vi "LinxDigitalRead.vi"(8 "Error In":errorcluster, 10 "Channels":u8[](array[numeric]), 11 "LINX Resource":T1) -> (0 "Error Out":errorcluster, 2 "Values":bool[](array[boolean]), 3 "LINX Resource":T1)   [LabVIEW 2020, in "LMH-LINX.lvlib" / "Local IO.lvlib"]
uses:
  Local IO.lvlib
  Type Defs/LINX Ref.ctl
  Type Defs/Platform.ctl
  Type Defs/Interface.ctl
  Device/Type Defs/LINX Device Config.ctl
  Device/Type Defs/TCP Config.ctl
  Device/Type Defs/Channels.ctl
  <vilib>/MakerHub/LINX/Resources/liblinxdevice.dll
  LMH-LINX.lvlib
  Device/Device.lvlib
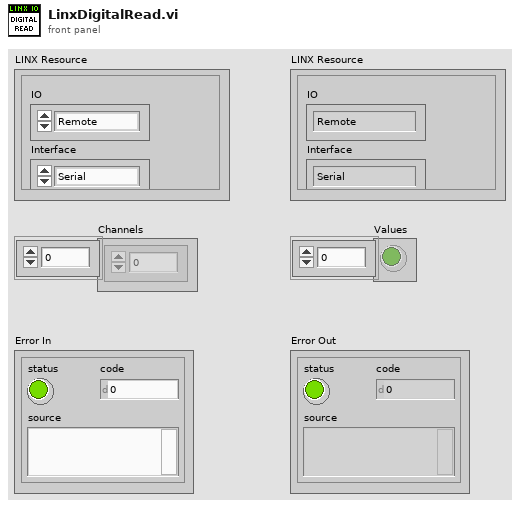
[diagram p1: front panel]
types:
  T1 = typedef "LMH-LINX.lvlib/LINX Ref.ctl" = cluster{"IO":T2, "Interface":T3, "LINX Device Config":T4}
  T2 = typedef "LMH-LINX.lvlib/Platform.ctl" = enum16{"Remote", "Local"}
  T3 = typedef "LMH-LINX.lvlib/Interface.ctl" = enum16{"Serial", "TCP"}
  T4 = typedef "LMH-LINX.lvlib/Device.lvlib/LINX Device Config.ctl" = cluster{"Interface":T3, "COM Port":refnum<visa-resource-name>, "TCP Configuration":T5, "Device Family":u8, "Device ID":u8, "Device Name":string, "TCP Ref":refnum<k5>, "Channels":T6}
  T5 = typedef "LMH-LINX.lvlib/Device.lvlib/TCP Config.ctl" = cluster{"IP Address":string, "Port":u16}
  T6 = typedef "LMH-LINX.lvlib/Channels.ctl" = cluster{"DI":u8[], "DO":u8[], "AI":u8[], "AO":u8[], "PWM":u8[], "QE":u8[], "UART":u8[], "I2C 2":u8[], "SPI":u8[], "CAN":u8[], "Servo":u8[], "AI Ref (V)":dbl, "AI Resolution (Bits)":u8, "AO Ref (V)":dbl, "AO Resolution (Bits)":u8}
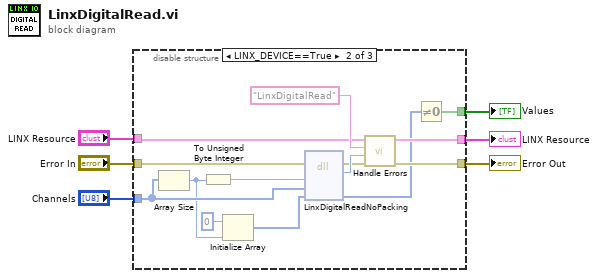
[diagram p0: block diagram]
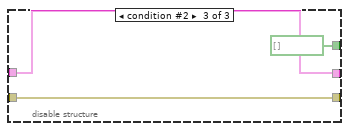
[diagram p3: hidden frame]
diagram:
  n1 = disable-structure shown="LINX_DEVICE==True" {
    disable-tunnel: [w8 w17 w24] -> w6
    disable-tunnel: [w7 w16 w25] -> w5
    disable-tunnel: "LINX Resource" -> [w8 w14 w24]
    disable-tunnel: "Error In" -> [w7 w15 w25]
    disable-tunnel: "Channels" -> [_ w13 _]
    disable-tunnel: [_ w9 bool[] [] ("Values")] -> w1
    frame condition #0 (active) {
    }
    frame condition #1 {
      n2 = Array Size(array=w13) -> (size(s)=w12:i32)
      n3 = To Unsigned Byte Integer(number=w12) -> (unsigned 8bit integer=w11:u8)
      n4 = Initialize Array(u8 0 ("element"), w12) -> (w22:u8[])
      n5 = dll-call lib="C:/Program Files (x86)/National Instruments/LabVIEW 2020/vi.lib/MakerHub/LINX/Resources/liblinxdevice.*" fn="LinxDigitalReadNoPacking"(error in=w15, "numChans"=w11, "channels"=w13, "values"=w22) -> (error out=w18:errorcluster, "LinxStatus"=w19:i32, "values"=w10:u8[])  [unwired: 4 in, 1 out]
      n6 = call <vilib>:"Handle Errors.vi"("Error In"=w18, "LinxStatus"=w19, "Function Name"="LinxDigitalRead", "LINX Resource"=w14) -> ("Error Out"=w16:errorcluster, "LINX Resource"=w17:T1)  [unwired: 6 in]
      n7 = Not Equal To 0?(x=w10) -> (x != 0?=w9:bool[])
    }
    frame condition #2 {
    }
  }
  "Error Out" <- w5
  "LINX Resource" <- w6
  "Values" <- w1
